vi "UHR-Fleezers Control (host) - 12.5.vi"() -> ()   [LabVIEW 2012] (continued)
            n2305 = Bundle("T1 Y", "T1 X", "T1 Sum", "T2 Y", "T2 X", "T2 Sum", "T1 FB X", "T1 FB Sum", "T2 FB X", "T2 FB Sum", "PSD Y", "PSD X", "PSD Y Sum") -> (w4151:T42)  [unwired: 1 out]
            n2306 = Cluster To Array(cluster=w4151) -> (array=w4160:string[])
          }
          frame "IR-QPD + PSD + FB-QPD XY positions" {
            w4225 = 4  # Channel pattern
            # "time average x2 the 3 psd signals (detection laser)"
            # "deinterlace 3 signals from qpds"
            n2307 = Decimate 1D Array(w4249) -> (w4248:i16[], w4247:i16[], w4226:i16[], w4246:i16[], w4192:i16[], w4238:i16[], w4237:i16[], w4214:i16[])
            n2308 = Decimate 1D Array "Feedback Sum"(w4226) -> (w4210:i16[], w4208:i16[])
            n2309 = Decimate 1D Array "QPD Y"(w4248) -> (w4245:i16[], w4228:i16[])
            n2310 = Decimate 1D Array "QPD X"(w4247) -> (w4244:i16[], w4242:i16[])
            n2311 = Decimate 1D Array "Feedback Y"(w4192) -> (w4191:i16[], w4190:i16[])
            n2312 = Decimate 1D Array "QPD Sum"(w4246) -> (w4243:i16[], w4241:i16[])
            n2313 = Decimate 1D Array "Feedback X"(w4214) -> (w4211:i16[], w4209:i16[])
            n2314 = call "downsample 1D array - double.vi"("Ave N"=2.0, "Array In"=w4238) -> ("Array Out"=w4213:dbl[])  [unwired: 1 out]
            n2315 = call "downsample 1D array - double.vi"("Ave N"=2.0, "Array In"=w4237) -> ("Array Out"=w4212:dbl[])  [unwired: 1 out]
            n2316 = Interleave 1D Arrays(w4245, w4244, w4243, w4228, w4242, w4241, w4191, w4211, w4210, w4190, w4209, w4208, w4213, w4212) -> (w4236:dbl[])
            n2317 = Divide(x=w4236, y=3276.7) -> (x/y=w4235:dbl[])
            n2318 = Decimate 1D Array(w4235) -> (w4234:dbl[], w4233:dbl[], w4232:dbl[], w4231:dbl[], w4230:dbl[], w4229:dbl[], w4187:dbl[], w4201:dbl[], w4185:dbl[], w4186:dbl[], w4199:dbl[], w4183:dbl[], w4197:dbl[], w4195:dbl[])
            n2319 = Negate(x=w4195) -> (-x=w4193:dbl[])
            n2320 = Divide(x=w4197, y=w4193) -> (x/y=w4196:dbl[])
            n2321 = Divide(x=w4186, y=w4183) -> (x/y=w4182:dbl[])
            n2322 = Divide(x=w4187, y=w4185) -> (x/y=w4184:dbl[])
            n2323 = Divide(x=w4234, y=w4232) -> (x/y=w4218:dbl[])
            n2324 = Divide(x=w4233, y=w4232) -> (x/y=w4217:dbl[])
            n2325 = Divide(x=w4231, y=w4229) -> (x/y=w4216:dbl[])
            n2326 = Divide(x=w4230, y=w4229) -> (x/y=w4215:dbl[])
            n2327 = Divide(x=w4201, y=w4185) -> (x/y=w4200:dbl[])
            n2328 = Divide(x=w4199, y=w4183) -> (x/y=w4198:dbl[])
            n2329 = Build Array(w4218, w4217, w4232, w4216, w4215, w4229, w4184, w4200, w4185, w4182, w4198, w4183, w4196, w4195) -> (w4194:dbl[][])
            n2330 = Bundle("T1 Y", "T1 X", "T1 Sum", "T2 Y", "T2 X", "T2 Sum", "T1 FB Y", "T1 FB X", "T1 FB Sum", "T2 FB Y", "T2 FB X", "T2 FB Sum", "PSD X", "PSD Y Sum") -> (w4181:T43)  [unwired: 1 out]
            n2331 = To Word Integer(number=w4236) -> (16bit integer=w4180:i16[])
            n2332 = Cluster To Array(cluster=w4181) -> (array=w4227:string[])
          }
        }
      }
    }
    "AI labels" <- w3250
    n2333 = local read "APD Integration Time (s)"() -> (w3223:dbl)
    n2334 = Array Size(array=w3265) -> (size(s)=w3310:i32)
    n2335 = call <vilib>:"Std Deviation and Variance.vi"("X"=w3212) -> ("standard deviation"=w3211:dbl)  [unwired: 1 in, 2 out]
    n2336 = Add Array Elements(numeric array=w3212) -> (sum=w3213:u32)
    n2337 = Add Array Elements(numeric array=w3265) -> (sum=w3320:u32)
    n2338 = call <vilib>:"Std Deviation and Variance.vi"("X"=w3265) -> ("standard deviation"=w3264:dbl)  [unwired: 1 in, 2 out]
    n2339 = Divide(x=w3211, y=w3053) -> (x/y=w3208:dbl)
    "Rate sigma (Hz) 2" <- w3208
    n2340 = Multiply(x=w3053, y=w3310) -> (x*y=w3055:dbl)
    "Int. Time (s)" <- w3055
    n2341 = Divide(x=w3213, y=w3055) -> (x/y=w3209:dbl)
    "APD 2 Rate (Hz)" <- w3209
    n2342 = Multiply(x="APD Disp. Scale", y=w3216) -> (x*y=w3225:waveform(dbl)[])
    n2343 = Divide(x=w3320, y=w3055) -> (x/y=w3262:dbl)
    "APD 1 Rate (Hz)" <- w3262
    n2344 = Divide(x=w3264, y=w3053) -> (x/y=w3263:dbl)
    "Rate sigma (Hz)" <- w3263
    n2345 = Divide(x=w3208, y=w3209) -> (x/y=→"Sigma/Mean 2":dbl)
    n2346 = Multiply(x="APD Disp. Downsample", y=w3223) -> (x*y=w3221:dbl)
    n2347 = Divide(x=w3263, y=w3262) -> (x/y=→"Sigma/Mean":dbl)
    n2348 = Divide(x=w3225, y=w3221) -> (x/y=w3045:waveform(dbl)[])
    n2349 = Index Array(array=w3045, index=0) -> (element=w3205:waveform(dbl))
    n2350 = Index Array(array=w3045, index=1) -> (element=w3203:waveform(dbl))
    n2351 = Index Array(array=w3045, index=2) -> (element=w3047:waveform(dbl))
    n2352 = Subtract(x=w3205, y="APD 1 Offset") -> (x-y=w3201:waveform(dbl))
    n2353 = Subtract(x=w3203, y="APD 2 Offset") -> (x-y=w3200:waveform(dbl))
    n2354 = Subtract(x=w3047, y="APD 3 Offset") -> (x-y=w3044:waveform(dbl))
    n2355 = Add Array Elements(numeric array=w3054) -> (sum=w3057:u32)
    n2356 = call <vilib>:"Std Deviation and Variance.vi"("X"=w3054) -> ("standard deviation"=w3056:dbl)  [unwired: 1 in, 2 out]
    n2357 = Build Array(w3201, w3200, w3044) -> (→"APD Chart":waveform(dbl)[])
    n2358 = Divide(x=w3057, y=w3055) -> (x/y=w3051:dbl)
    "APD 3 Rate (Hz)" <- w3051
    n2359 = Divide(x=w3056, y=w3053) -> (x/y=w3052:dbl)
    "Rate sigma (Hz) 3" <- w3052
    n2360 = Divide(x=w3052, y=w3051) -> (x/y=→"Sigma/Mean 3":dbl)
    n2361 = local read "Data Period (s)"() -> (w3108:dbl)
    n2362 = local read "BD 1 Frequency 2 (MHz)"() -> (w3141:dbl)
    n2363 = local read "BD 1 Frequency 1 (MHz)"() -> (w3142:dbl)
    n2364 = Decimate 1D Array(w3149) -> (w3173:i16[], w3172:i16[], w3170:i16[], w3169:i16[])  [unwired: 9 out]
    n2365 = Multiply(x=w3108, y="Trap Pos. Disp. Downsample") -> (x*y=w3106:dbl)
    n2366 = Divide(x=w3173, y=w3172) -> (x/y=w3174:dbl[])
    n2367 = Divide(x=w3170, y=w3169) -> (x/y=w3171:dbl[])
    n2368 = local read "AOM X Cal (nm/MHz)"() -> (w3139:dbl)
    n2369 = Split 1D Array(array=w3174, index="N El. to Ave.") -> (second subarray=w3177:dbl[])  [unwired: 1 out]
    n2370 = Split 1D Array(array=w3171, index="N El. to Ave.") -> (second subarray=w3176:dbl[])  [unwired: 1 out]
    n2371 = Multiply(x=w3108, y="Trap Disp. Downsample") -> (x*y=w3187:dbl)
    "Display Period (s)" <- w3187
    n2372 = for "Trap AI" {
      tunnel: [w3974] -> w3352 mode=indexing
      tunnel: w3185 -> [w3965]
      tunnel: "Trap Disp. Downsample" -> [w3972]
      tunnel: w3251 -> [w3970] mode=indexing
      tunnel: w3108 -> [w3969]
      tunnel: w3250 -> [w3968] mode=indexing
      tunnel: [w3967] -> w3220 mode=indexing
      tunnel: w3187 -> [w3966]
      workers-P: _ -> [_]
      n2373 = Bundle By Name("Y"=w3970, "dt"=w3969) -> (w3971:waveform(dbl))  [unwired: 1 out]
      n2374 = Set Waveform Attribute(5:w3968, 6:"NI_ChannelName" ("name"), 7:w3971) -> (3:w3967:waveform(dbl))  [unwired: 1 in, 2 out]
      n2375 = call "downsample 1D array - double.vi"("Ave N"=w3972, "Array In"=w3970) -> ("Array Out"=w3973:dbl[])  [unwired: 1 out]
      n2376 = Bundle By Name(cluster=w3967, "t0"=w3965, "Y"=w3973, "dt"=w3966) -> (w3974:waveform(dbl))
    }
    n2377 = Bundle("BD 1 Frequency 1 (MHz)"=w3142, "BD 1 Frequency 2 (MHz)"=w3141) -> (w3143:T44)  [unwired: 1 out]
    n2378 = call-poly <vilib>:"Mean.vi"("X"=w3176) -> ("mean"=w3164:dbl)  [unwired: 1 out]
    n2379 = call-poly <vilib>:"Mean.vi"("X"=w3177) -> ("mean"=w3165:dbl)  [unwired: 1 out]
    n2380 = Reciprocal(x=w3187) -> (1/x=→"Trap Disp. Freq. (Hz)":dbl)
    n2381 = Cluster To Array(cluster=w3143) -> (array=w3140:dbl[])
    n2382 = local read "Trap X AI1 (DMA)"() -> (w3175:T13)
    n2383 = local read "Data points/scans (MCL)"() -> (w3330:dbl)
    n2384 = To Fixed-Point(number=w3164) -> (fixed-point=w3162:fxp<+/-,16,1>)  [unwired: 1 in]
    n2385 = To Fixed-Point(number=w3165) -> (fixed-point=w3163:fxp<+/-,16,1>)  [unwired: 1 in]
    n2386 = Bundle("Trap 1 Pos.", "Trap 2 Pos.") -> (w3184:cluster{string, string})  [unwired: 1 out]
    n2387 = Bundle By Name(cluster=w3175, "Set 1"=w3163, "Set 2"=w3162) -> (→"Trap X AI1 (DMA)":T13)
    n2388 = Cluster To Array(cluster=w3184) -> (array=w3181:string[])
    n2389 = Unbundle(w3041) -> (w3042:u32[])  [unwired: 2 out]
    n2390 = Select(t=-1.0, s="Negate Y Axis", f=1.0) -> (s? t:f=w3125:dbl)
    n2391 = for "Trap Position" {
      tunnel: w3189 -> [w3560] mode=indexing
      tunnel: "Trap Pos. Disp. Downsample" -> [w3559]
      tunnel: w3106 -> [w3557]
      tunnel: w3185 -> [w3556]
      tunnel: w3181 -> [w3554] mode=indexing
      tunnel: [w3553] -> w3095 mode=indexing
      tunnel: w3140 -> [w3551] mode=indexing
      tunnel: w3139 -> [w3549]
      tunnel: w3125 -> [w3548]
      n2392 = call "downsample 1D array - double.vi"("Ave N"=w3559, "Array In"=w3560) -> ("Array Out"=w3558:dbl[])  [unwired: 1 out]
      n2393 = Subtract(x=w3558, y=w3551) -> (x-y=w3552:dbl[])
      n2394 = Multiply(x=w3549, y=w3552) -> (x*y=w3550:dbl[])
      n2395 = Multiply(x=w3548, y=w3550) -> (x*y=w3547:dbl[])
      n2396 = Bundle By Name("Y"=w3547, "dt"=w3557, "t0"=w3556) -> (w3555:waveform(dbl))  [unwired: 1 out]
      n2397 = Set Waveform Attribute(5:w3554, 6:"NI_ChannelName" ("name"), 7:w3555) -> (3:w3553:waveform(dbl))  [unwired: 1 in, 2 out]
    }
    n2398 = To Double Precision Float(number=w3042) -> (double precision float=w3248:dbl[])
    n2399 = local read "Display Period (s)"() -> (w3237:dbl)
    n2400 = Increment(x=w3330) -> (x+1=w3331:dbl)
    n2401 = Index Array(array=w3095, index=0) -> (element=w3099:waveform(dbl))
    n2402 = Index Array(array=w3095, index=1) -> (element=w3094:waveform(dbl))
    n2403 = feedback #7(w3331) -> (w3334:dbl)
    n2404 = Select(t=0, s=w3321, f=w3334) -> (s? t:f=w3327:dbl)
    n2405 = Array Size(array=w3248) -> (size(s)=w3333:i32)
    n2406 = Build Array (concatenate)(w3216, w3352) -> (w3218:waveform(dbl)[])
    "All Signals" <- w3218
    n2407 = Add(x=w3333, y=w3327) -> (x+y=w3328:dbl)
    n2408 = Unbundle By Name(w3099) -> ("Y"=w3100:dbl[])
    n2409 = Divide(x="Bead Sep. Int. Time (s)", y=w3237) -> (x/y=w3135:dbl)
    n2410 = Add(x=w3100, y="FB Trap Pos Offset") -> (x+y=w3098:dbl[])
    "T1 x pos data" <- w3098
    n2411 = Greater?(x=w3328, y=w3330) -> (0:w3329:bool)
    n2412 = feedback #8(w3098) -> (w3137:dbl[])
    n2413 = Build Array (concatenate)(w3098, w3137) -> (w3136:dbl[])
    n2414 = Bundle By Name(cluster=w3099, "Y"=w3098) -> (w3097:waveform(dbl))
    n2415 = Select(t=w3327, s=w3329, f=w3328) -> (s? t:f=w3326:dbl)
    n2416 = feedback-in #7(w3326) -> ()
    n2417 = local read "MCL Scanning"() -> (w3324:bool)
    n2418 = Bundle(w3097, w3094) -> (w3093:cluster{waveform(dbl), waveform(dbl)})  [unwired: 1 out]
    n2419 = Split 1D Array(array=w3136, index=w3135) -> (first subarray=w3129:dbl[])  [unwired: 1 out]
    n2420 = feedback-in #8(w3129) -> ()
    n2421 = Not(x=w3329) -> (.not. x?=w3323:bool)
    n2422 = Cluster To Array(cluster=w3093) -> (array=w3069:waveform(dbl)[])
    "Trap Positions" <- w3069
    n2423 = call-poly <vilib>:"Mean.vi"("X"=w3129) -> ("mean"=w3128:dbl)  [unwired: 1 out]
    "Mean T1 Position (nm)" <- w3128
    n2424 = Subtract(x=w3129, y=w3128) -> (x-y=w3134:dbl[])
    n2425 = Square(x=w3134) -> (x^2=w3133:dbl[])
    n2426 = And(x=w3323, y=w3324) -> (x .and. y?=w3325:bool)
    n2427 = call-poly <vilib>:"Mean.vi"("X"=w3133) -> ("mean"=w3132:dbl)  [unwired: 1 out]
    n2428 = Square Root(x=w3132) -> (sqrt(x)=w3131:dbl)
    n2429 = Or(x=w3325, y=w3321) -> (x .or. y?=w3322:bool)
    n2430 = Equal?(x="Tab Control 6", y=T34."High Res Display") -> (x = y?=w3254:bool)
    n2431 = Multiply(x=10.0, y=w3131) -> (x*y=→"Trap 1 Position RMS (A)":dbl)
    n2432 = case "For displaying the high resolution display (no downsampling)" shown="True" w3254 {
      tunnel: w3220 -> [_ w3580]
      frame False {
      }
      frame True {
        n2433 = Index Array(array=w3580, index="High Res. Display") -> (element=w3581:waveform(dbl))
        n2434 = call <vilib>:"Std Deviation and Variance.vi"("X"=w3581) -> ("mean"=w3588:dbl, "standard deviation"=w3593:dbl)  [unwired: 1 in, 1 out]
        "Mean Intensity" <- w3588
        "Sigma" <- w3593
        n2435 = Subtract(x=w3581, y=w3588) -> (x-y=w3587:waveform(dbl))
        n2436 = Select(t=w3587, s="Subtract mean", f=w3581) -> (s? t:f=→"1 Channel":waveform(dbl))
        n2437 = Divide(x=w3593, y=w3588) -> (x/y=→"Sigma/Mean":dbl)
        n2438 = feedback #9(1) -> (w3582:i32)
        n2439 = Greater Or Equal?(x=w3582, y="Slow mean N ave.") -> (x >= y?=w3595:bool)
        n2440 = Increment(x=w3582) -> (x+1=w3597:i32)
        n2441 = Select(t=1, s=w3595, f=w3597) -> (s? t:f=w3584:i32)
        n2442 = feedback-in #9(w3584) -> ()
        n2443 = feedback #10() -> (w3585:waveform(dbl))  [unwired: 1 out]
        n2444 = case shown="Default" w3582 {
          tunnel: [w3600 w3603] -> w3586
          tunnel: w3585 -> [w3602 _]
          tunnel: w3581 -> [w3601 w3603]
          frame Default {
            n2445 = call-poly <vilib>:"Append Waveforms.vi"("waveform B"=w3601, "waveform A"=w3602) -> ("waveform out"=w3600:waveform(dbl))  [unwired: 1 in, 8 out]
          }
          frame 1 {
          }
        }
        n2446 = feedback-in #10(w3586) -> ()
        n2447 = case shown="True" w3595 {
          tunnel: w3586 -> [_ w3599]
          frame False {
          }
          frame True {
            n2448 = call-poly <vilib>:"Mean.vi"("X"=w3599) -> ("mean"=→"Slow mean":dbl)  [unwired: 1 out]
          }
        }
      }
    }
    n2449 = case "For plotting results of scanning MCL (fluorescence and detection laser images)" shown="True" w3322 {
      tunnel: w3321 -> [_ w3712]
      tunnel: w3330 -> [_ _]
      tunnel: w3220 -> [_ w3842]
      tunnel: w3198 -> [_ w3750]
      tunnel: w3041 -> [_ w3719]
      frame False {
      }
      frame True {
        w3729 = u32 0 items=["Horizontal", "Vertical", "Central", "1st Diagonal", "2nd Diagonal"] ("Type of Symmetry")
        w3757 = u32 0 items=["Horizontal", "Vertical", "Central", "1st Diagonal", "2nd Diagonal"] ("Type of Symmetry")
        w3781 = u32 0 items=["Horizontal", "Vertical", "Central", "1st Diagonal", "2nd Diagonal"] ("Type of Symmetry")
        w3784 = u32 0 items=["Horizontal", "Vertical", "Central", "1st Diagonal", "2nd Diagonal"] ("Type of Symmetry")
        w3813 = u32 0 items=["Horizontal", "Vertical", "Central", "1st Diagonal", "2nd Diagonal"] ("Type of Symmetry")
        n2450 = Unbundle(w3719) -> (w3718:u32[], w3716:u32[], w3714:u32[])
        n2451 = To Double Precision Float(number=w3718) -> (double precision float=w3717:dbl[])
        n2452 = To Double Precision Float(number=w3716) -> (double precision float=w3715:dbl[])
        n2453 = To Double Precision Float(number=w3714) -> (double precision float=w3713:dbl[])
        n2454 = Index Array(array=w3842, index=10) -> (element=w3848:waveform(dbl))
        n2455 = Index Array(array=w3842, index=11) -> (element=w3845:waveform(dbl))
        n2456 = local read "Cycles/step (MCL)"() -> (w3798:u64)
        n2457 = Index Array(array=w3842, index="Channel") -> (element=w3844:waveform(dbl))
        n2458 = Unbundle(w3750) -> ("New Image"=w3749:T2, "New Image"=w3748:T2, "New Image"=w3720:T2, "New Image"=w3721:T2, "New Image"=w3722:T2)
        n2459 = local read "Scan steps (MCL)"() -> (w3708:u64)
        n2460 = Unbundle By Name(w3848) -> ("Y"=w3800:dbl[])
        n2461 = Unbundle By Name(w3845) -> ("Y"=w3802:dbl[])
        n2462 = local read "Scan lines (y)"() -> (w3709:u64)
        n2463 = local read "N APD Samp/step"() -> (w3711:dbl)
        n2464 = Unbundle By Name(w3844) -> ("Y"=w3807:dbl[])
        n2465 = call "downsample 1D array - double.vi"("Ave N"=w3798, "Array In"=w3800) -> ("Array Out"=w3799:dbl[])  [unwired: 1 out]
        n2466 = call "downsample 1D array - double.vi"("Ave N"=w3798, "Array In"=w3802) -> ("Array Out"=w3801:dbl[])  [unwired: 1 out]
        n2467 = call "downsample 1D array - double.vi"("Ave N"=w3798, "Array In"=w3807) -> ("Array Out"=w3806:dbl[])  [unwired: 1 out]
        n2468 = Multiply(x=w3708, y=u64 2) -> (x*y=w3710:u64)
        n2469 = feedback #11(w3715) -> (w3775:dbl[])
        n2470 = Build Array (concatenate)(w3775, w3715) -> (w3774:dbl[])
        n2471 = feedback #12(w3713) -> (w3747:dbl[])
        n2472 = Build Array (concatenate)(w3747, w3713) -> (w3746:dbl[])
        n2473 = Select(t=w3715, s=w3712, f=w3774) -> (s? t:f=w3759:dbl[])
        n2474 = feedback-in #11(w3759) -> ()
        n2475 = Select(t=w3713, s=w3712, f=w3746) -> (s? t:f=w3731:dbl[])
        n2476 = feedback-in #12(w3731) -> ()
        n2477 = feedback #13(w3717) -> (w3868:dbl[])
        n2478 = Build Array (concatenate)(w3868, w3717) -> (w3850:dbl[])
        n2479 = Select(t=w3717, s=w3712, f=w3850) -> (s? t:f=w3854:dbl[])
        n2480 = feedback-in #13(w3854) -> ()
        n2481 = feedback #14(w3799) -> (w3856:dbl[])
        n2482 = Build Array (concatenate)(w3856, w3799) -> (w3847:dbl[])
        n2483 = feedback #15(w3806) -> (w3866:dbl[])
        n2484 = Build Array (concatenate)(w3866, w3806) -> (w3865:dbl[])
        n2485 = feedback #16(w3801) -> (w3858:dbl[])
        n2486 = Build Array (concatenate)(w3858, w3801) -> (w3859:dbl[])
        n2487 = Select(t=w3799, s=w3712, f=w3847) -> (s? t:f=w3803:dbl[])
        n2488 = feedback-in #14(w3803) -> ()
        n2489 = Select(t=w3806, s=w3712, f=w3865) -> (s? t:f=w3805:dbl[])
        n2490 = feedback-in #15(w3805) -> ()
        n2491 = Select(t=w3801, s=w3712, f=w3859) -> (s? t:f=w3804:dbl[])
        n2492 = feedback-in #16(w3804) -> ()
        n2493 = call "integrate 1D array interval - double.vi"("Ave N"=w3711, "Array In"=w3759) -> ("Array Out"=w3770:dbl[])  [unwired: 1 out]
        n2494 = call "integrate 1D array interval - double.vi"("Ave N"=w3711, "Array In"=w3731) -> ("Array Out"=w3742:dbl[])  [unwired: 1 out]
        n2495 = call "integrate 1D array interval - double.vi"("Ave N"=w3711, "Array In"=w3854) -> ("Array Out"=w3853:dbl[])  [unwired: 1 out]
        n2496 = Array Size(array=w3770) -> (size(s)=w3771:i32)
        n2497 = Array Size(array=w3742) -> (size(s)=w3743:i32)
        n2498 = Array Size(array=w3853) -> (size(s)=w3855:i32)
        n2499 = Multiply(x=w3709, y=w3710) -> (x*y=w3773:u64)
        n2500 = Multiply(x=w3709, y=w3710) -> (x*y=w3745:u64)
        n2501 = Multiply(x=w3709, y=w3710) -> (x*y=w3863:u64)
        n2502 = Subtract(x=w3773, y=w3771) -> (x-y=w3764:u64)
        n2503 = call-poly <vilib>:"Mean.vi"("X"=w3770) -> ("mean"=w3761:dbl)  [unwired: 1 out]
        n2504 = Subtract(x=w3745, y=w3743) -> (x-y=w3736:u64)
        n2505 = call-poly <vilib>:"Mean.vi"("X"=w3742) -> ("mean"=w3733:dbl)  [unwired: 1 out]
        n2506 = Subtract(x=w3863, y=w3855) -> (x-y=w3797:u64)
        n2507 = call-poly <vilib>:"Mean.vi"("X"=w3853) -> ("mean"=w3794:dbl)  [unwired: 1 out]
        n2508 = call-poly <vilib>:"Mean.vi"("X"=w3803) -> ("mean"=w3787:dbl)  [unwired: 1 out]
        n2509 = call-poly <vilib>:"Mean.vi"("X"=w3805) -> ("mean"=w3792:dbl)  [unwired: 1 out]
        n2510 = call-poly <vilib>:"Mean.vi"("X"=w3804) -> ("mean"=w3790:dbl)  [unwired: 1 out]
        n2511 = Initialize Array(1.0 ("element"), w3764) -> (w3760:dbl[])
        n2512 = Initialize Array(1.0 ("element"), w3736) -> (w3732:dbl[])
        n2513 = Initialize Array(1.0 ("element"), w3797) -> (w3788:dbl[])
        n2514 = Multiply(x=w3760, y=w3761) -> (x*y=w3762:dbl[])
        n2515 = Multiply(x=w3732, y=w3733) -> (x*y=w3734:dbl[])
        n2516 = Multiply(x=w3788, y=w3794) -> (x*y=w3795:dbl[])
        n2517 = Multiply(x=w3788, y=w3790) -> (x*y=w3791:dbl[])
        n2518 = Multiply(x=w3788, y=w3792) -> (x*y=w3793:dbl[])
        n2519 = Multiply(x=w3788, y=w3787) -> (x*y=w3789:dbl[])
        n2520 = Build Array (concatenate)(w3770, w3762) -> (w3772:dbl[])
        n2521 = Build Array (concatenate)(w3742, w3734) -> (w3744:dbl[])
        n2522 = Build Array (concatenate)(w3853, w3795) -> (w3862:dbl[])
        n2523 = Build Array (concatenate)(w3803, w3789) -> (w3857:dbl[])
        n2524 = Build Array (concatenate)(w3805, w3793) -> (w3861:dbl[])
        n2525 = Build Array (concatenate)(w3804, w3791) -> (w3860:dbl[])
        n2526 = Reshape Array(w3772, w3709, w3710) -> (w3768:dbl[][])
        n2527 = Reshape Array(w3744, w3709, w3710) -> (w3740:dbl[][])
        n2528 = Reshape Array(w3862, w3709, w3710) -> (w3840:dbl[][])
        n2529 = Reshape Array(w3857, w3709, w3710) -> (w3823:dbl[][])
        n2530 = Reshape Array(w3861, w3709, w3710) -> (w3815:dbl[][])
        n2531 = Reshape Array(w3860, w3709, w3710) -> (w3830:dbl[][])
        n2532 = Array Subset(array=w3768, index (col)=0 ("index"), length (col)=w3708) -> (w3767:dbl[][])  [unwired: 2 in]
        n2533 = Array Subset(array=w3768, index (col)=w3708) -> (w3765:dbl[][])  [unwired: 3 in]
        n2534 = Array Subset(array=w3740, index (col)=0 ("index"), length (col)=w3708) -> (w3739:dbl[][])  [unwired: 2 in]
        n2535 = Array Subset(array=w3740, index (col)=w3708) -> (w3737:dbl[][])  [unwired: 3 in]
        n2536 = Array Subset(array=w3830, index (col)=0 ("index"), length (col)=w3708) -> (w3835:dbl[][])  [unwired: 2 in]
        n2537 = Array Subset(array=w3830, index (col)=w3708) -> (w3833:dbl[][])  [unwired: 3 in]
        n2538 = Array Subset(array=w3840, index (col)=0 ("index"), length (col)=w3708) -> (w3839:dbl[][])  [unwired: 2 in]
        n2539 = Array Subset(array=w3840, index (col)=w3708) -> (w3837:dbl[][])  [unwired: 3 in]
        n2540 = Array Subset(array=w3815, index (col)=0 ("index"), length (col)=w3708) -> (w3821:dbl[][])  [unwired: 2 in]
        n2541 = Array Subset(array=w3815, index (col)=w3708) -> (w3819:dbl[][])  [unwired: 3 in]
        n2542 = Array Subset(array=w3823, index (col)=0 ("index"), length (col)=w3708) -> (w3828:dbl[][])  [unwired: 2 in]
        n2543 = Array Subset(array=w3823, index (col)=w3708) -> (w3826:dbl[][])  [unwired: 3 in]
        n2544 = for {
          tunnel: w3767 -> [w3872] mode=indexing
          tunnel: [w3871] -> w3766 mode=indexing
          workers-P: _ -> [_]
          n2545 = Reverse 1D Array(array=w3872) -> (reversed array=w3871:dbl[])
        }
        n2546 = for {
          tunnel: w3739 -> [w3870] mode=indexing
          tunnel: [w3869] -> w3738 mode=indexing
          workers-P: _ -> [_]
          n2547 = Reverse 1D Array(array=w3870) -> (reversed array=w3869:dbl[])
        }
        n2548 = for {
          tunnel: w3835 -> [w3878] mode=indexing
          tunnel: [w3877] -> w3834 mode=indexing
          workers-P: _ -> [_]
          n2549 = Reverse 1D Array(array=w3878) -> (reversed array=w3877:dbl[])
        }
        n2550 = for {
          tunnel: w3839 -> [w3880] mode=indexing
          tunnel: [w3879] -> w3838 mode=indexing
          workers-P: _ -> [_]
          n2551 = Reverse 1D Array(array=w3880) -> (reversed array=w3879:dbl[])
        }
        n2552 = for {
          tunnel: w3821 -> [w3874] mode=indexing
          tunnel: [w3873] -> w3820 mode=indexing
          workers-P: _ -> [_]
          n2553 = Reverse 1D Array(array=w3874) -> (reversed array=w3873:dbl[])
        }
        n2554 = for {
          tunnel: w3828 -> [w3876] mode=indexing
          tunnel: [w3875] -> w3827 mode=indexing
          workers-P: _ -> [_]
          n2555 = Reverse 1D Array(array=w3876) -> (reversed array=w3875:dbl[])
        }
        n2556 = Index Array(array=w3840, index (row)=0) -> (element=→"Waveform Graph":dbl[])  [unwired: 1 in]
        n2557 = Add(x=w3766, y=w3765) -> (x+y=w3752:dbl[][])
        n2558 = Add(x=w3738, y=w3737) -> (x+y=w3724:dbl[][])
        n2559 = Add(x=w3834, y=w3833) -> (x+y=w3832:dbl[][])
        n2560 = Add(x=w3838, y=w3837) -> (x+y=w3812:dbl[][])
        n2561 = Add(x=w3820, y=w3819) -> (x+y=w3818:dbl[][])
        n2562 = Add(x=w3827, y=w3826) -> (x+y=w3825:dbl[][])
        n2563 = Divide(x=w3818, y=2) -> (x/y=w3816:dbl[][])
        n2564 = Divide(x=w3832, y=2) -> (x/y=w3777:dbl[][])
        n2565 = To Single Precision Float(number=w3812) -> (single precision float=w3811:sgl[][])
        n2566 = To Single Precision Float(number=w3752) -> (single precision float=w3756:sgl[][])
        n2567 = To Single Precision Float(number=w3724) -> (single precision float=w3728:sgl[][])
        n2568 = Divide(x=w3825, y=2) -> (x/y=w3779:dbl[][])
        n2569 = Transpose 2D Array(2D array=w3816) -> (transposed array=→"Data map":dbl[][])
        n2570 = To Single Precision Float(number=w3777) -> (single precision float=w3783:sgl[][])
        n2571 = To Single Precision Float(number=w3779) -> (single precision float=w3780:sgl[][])
        n2572 = call "IMAQ ArrayToImage"("Image Pixels (Float)"=w3811, "Image"=w3749) -> ("Image Out"=w3814:T2)  [unwired: 8 in, 1 out]
        n2573 = call "IMAQ ArrayToImage"("Image Pixels (Float)"=w3756, "Image"=w3748) -> ("Image Out"=w3758:T2)  [unwired: 8 in, 1 out]
        n2574 = call "IMAQ ArrayToImage"("Image Pixels (Float)"=w3728, "Image"=w3720) -> ("Image Out"=w3730:T2)  [unwired: 8 in, 1 out]
        n2575 = call "IMAQ ArrayToImage"("Image Pixels (Float)"=w3783, "Image"=w3721) -> ("Image Out"=w3785:T2)  [unwired: 8 in, 1 out]
        n2576 = call "IMAQ Symmetry"("Type of Symmetry"=w3813, "Image Src"=w3814) -> ("Image Dst Out"=w3809:T2)  [unwired: 3 in, 1 out]
        n2577 = call "IMAQ ArrayToImage"("Image Pixels (Float)"=w3780, "Image"=w3722) -> ("Image Out"=w3782:T2)  [unwired: 8 in, 1 out]
        n2578 = call "IMAQ Symmetry"("Type of Symmetry"=w3757, "Image Src"=w3758) -> ("Image Dst Out"=w3754:T2)  [unwired: 3 in, 1 out]
        n2579 = call "IMAQ Symmetry"("Type of Symmetry"=w3729, "Image Src"=w3730) -> ("Image Dst Out"=w3726:T2)  [unwired: 3 in, 1 out]
        n2580 = call "IMAQ Symmetry"("Type of Symmetry"=w3784, "Image Src"=w3785) -> ("Image Dst Out"=→"Detection Laser X":T2)  [unwired: 3 in, 1 out]
        n2581 = call "IMAQ Symmetry"("Type of Symmetry"=w3781, "Image Src"=w3782) -> ("Image Dst Out"=→"Detection Laser Y":T2)  [unwired: 3 in, 1 out]
        n2582 = call "IMAQ Set Simple Calibration"("Calibration Axis Info"=T35 {"Origin Pixel"={"X"=0.0, "Y"=0.0}, "Angle Relative to Horizontal (deg)"=0.0, "Axis Reference"=0}, "Grid Descriptor"=T36 {"X Step"=0.3, "Y Step"=0.3, "Unit"=enum."Undefined"}, "Image"=w3809) -> ("Calibrated Image"=→"APD 1":T2)  [unwired: 7 in, 1 out]
        n2583 = call "IMAQ Set Simple Calibration"("Calibration Axis Info"=T35 {"Origin Pixel"={"X"=0.0, "Y"=0.0}, "Angle Relative to Horizontal (deg)"=0.0, "Axis Reference"=0}, "Grid Descriptor"=T36 {"X Step"=0.3, "Y Step"=0.3, "Unit"=enum."Undefined"}, "Image"=w3754) -> ("Calibrated Image"=→"APD 2":T2)  [unwired: 7 in, 1 out]
        n2584 = call "IMAQ Set Simple Calibration"("Calibration Axis Info"=T35 {"Origin Pixel"={"X"=0.0, "Y"=0.0}, "Angle Relative to Horizontal (deg)"=0.0, "Axis Reference"=0}, "Grid Descriptor"=T36 {"X Step"=0.3, "Y Step"=0.3, "Unit"=enum."Undefined"}, "Image"=w3726) -> ("Calibrated Image"=→"APD 3":T2)  [unwired: 7 in, 1 out]
      }
    }
    n2585 = case "For computing FFTs for display" shown="True" "Compute FFT" {
      tunnel: w3220 -> [_ w4352]
      frame False {
      }
      frame True {
        n2586 = Build Array("FFT 1 Choice 1", "FFT 1 Choice 2", "FFT 2 Choice 1", "FFT 2 Choice 2") -> (w4345:u16[])
        n2587 = Array Size(array=w4352) -> (size(s)=w4351:i32)
        n2588 = feedback-in #17(w4345) -> ()
        n2589 = feedback #17(u16[] [100, 100, 100, 100]) -> (w4346:u16[])
        n2590 = feedback-in #18("# Spectra to Ave.") -> ()
        n2591 = feedback #18("# Spectra to Ave.") -> (w4343:dbl)
        n2592 = Not Equal?(x="# Spectra to Ave.", y=w4343) -> (x != y?=w4342:bool)
        n2593 = Not Equal?(x=w4345, y=w4346) -> (x != y?=w4344:bool)
        n2594 = feedback #19(1.0) -> (w4329:dbl)
        n2595 = Compound Arithmetic op=OR("Reset FFT", w4344, w4342) -> (w4327:bool)
        n2596 = Select(t=1.0, s=w4327, f=w4329) -> (s? t:f=w4331:dbl)
        n2597 = Greater?(x=w4331, y="# Spectra to Ave.") -> (0:w4350:bool)
        n2598 = Increment(x=w4331) -> (x+1=w4330:dbl)
        n2599 = feedback-in #19(w4330) -> ()
        n2600 = local read "DMA Update Period (s)"() -> (w4325:dbl)
        n2601 = Multiply(x="# Spectra to Ave.", y=w4325) -> (x*y=→"Ave. Time (s)":dbl)
        n2602 = Build Array(cluster{"f0":dbl, "df":dbl, "magnitude":dbl[]} {"f0"=0.0, "df"=0.0, "magnitude"=[]} ("PSD")) -> (w4334:cluster{"f0":dbl, "df":dbl, "magnitude":dbl[]}[])
        n2603 = Build Array(w4334, w4334, w4334, w4334) -> (w4336:T45)
        n2604 = feedback #20(w4336) -> (w4341:T45)
        n2605 = for {
          N: 4 -> [_]
          tunnel: w4345 -> [w4374] mode=indexing
          tunnel: w4352 -> [w4375]
          tunnel: w4351 -> [w4377]
          tunnel: w4327 -> [w4370]
          tunnel: w4350 -> [w4369]
          tunnel: "# Spectra to Ave." -> [w4368]
          tunnel: [w4367] -> w4340 mode=indexing
          tunnel: w4341 -> [w4372] mode=indexing
          tunnel: [w4371] -> w4328 mode=indexing
          tunnel: w4331 -> [w4366]
          n2606 = Less?(x=w4374, y=w4377) -> (x < y?=w4376:bool)
          n2607 = Index Array(array=w4375, index=w4374) -> (element=w4373:waveform(dbl))
          n2608 = case shown="True" w4376 {
            tunnel: w4373 -> [_ w4394]
            tunnel: w4372 -> [w4379 w4392]
            tunnel: [w4379 w4380] -> w4371
            tunnel: w4370 -> [_ w4391]
            tunnel: w4369 -> [_ w4384]
            tunnel: w4368 -> [_ w4383]
            tunnel: [cluster{"f0":dbl, "df":dbl, "magnitude":dbl[]} {"f0"=0.0, "df"=0.0, "magnitude"=[]} ("PSD") w4385] -> w4367
            tunnel: w4366 -> [_ w4382]
            frame False {
            }
            frame True {
              n2609 = call <vilib>:"Std Deviation and Variance.vi"("X"=w4394) -> ("mean"=w4395:dbl)  [unwired: 1 in, 2 out]
              n2610 = Subtract(x=w4394, y=w4395) -> (x-y=w4393:waveform(dbl))
              n2611 = xnode "Spectral Measurements"("Signals"=w4393) -> ("PSD"=w4387:cluster{"f0":dbl, "df":dbl, "magnitude":dbl[]})  [unwired: 1 in, 1 out]
              n2612 = case shown="False" w4391 {
                tunnel: w4392 -> [w4404 _]
                tunnel: [w4400 w4409] -> w4380
                tunnel: w4387 -> [w4403 w4410]
                tunnel: w4384 -> [w4402 _]
                frame False {
                  n2613 = Build Array (concatenate)(w4404, w4403) -> (w4401:cluster{"f0":dbl, "df":dbl, "magnitude":dbl[]}[])
                  n2614 = case shown="True" w4402 {
                    tunnel: w4401 -> [w4405 w4408]
                    tunnel: [w4405 w4406] -> w4400
                    frame False {
                    }
                    frame True {
                      n2615 = Delete From Array(array=w4408, index=0) -> (array with subset deleted=w4406:cluster{"f0":dbl, "df":dbl, "magnitude":dbl[]}[])  [unwired: 1 in, 1 out]
                    }
                  }
                }
                frame True {
                  n2616 = Build Array(w4410) -> (w4409:cluster{"f0":dbl, "df":dbl, "magnitude":dbl[]}[])
                }
              }
              n2617 = for {
                tunnel: w4380 -> [w4399] mode=indexing
                tunnel: [w4398] -> w4390 mode=indexing
                workers-P: _ -> [_]
                n2618 = Unbundle By Name(w4399) -> ("magnitude"=w4398:dbl[])
              }
              n2619 = Transpose 2D Array(2D array=w4390) -> (transposed array=w4389:dbl[][])
              n2620 = for {
                tunnel: w4389 -> [w4397] mode=indexing
                tunnel: [w4396] -> w4388 mode=indexing
                workers-P: _ -> [_]
                n2621 = Add Array Elements(numeric array=w4397) -> (sum=w4396:dbl)
              }
              n2622 = Select(t=w4383, s=w4384, f=w4382) -> (s? t:f=w4381:dbl)
              n2623 = Divide(x=w4388, y=w4381) -> (x/y=w4386:dbl[])
              n2624 = Bundle By Name(cluster=w4387, "magnitude"=w4386) -> (w4385:cluster{"f0":dbl, "df":dbl, "magnitude":dbl[]})
            }
          }
        }
        n2625 = case shown="True" w4327 {
          tunnel: w4328 -> [w4359 w4365]
          tunnel: [w4359 w4360] -> w4326
          frame False {
          }
          frame True {
            n2626 = Array Subset(array=w4365, index (row)=0 ("index"), length (row)=4 ("length"), index (col)=0 ("index"), length (col)=1 ("length")) -> (w4360:T45)
          }
        }
        n2627 = feedback-in #20(w4326) -> ()
        n2628 = Split 1D Array(array=w4340, index=2) -> (first subarray=→"FFT 1":cluster{"f0":dbl, "df":dbl, "magnitude":dbl[]}[], second subarray=→"FFT 2":cluster{"f0":dbl, "df":dbl, "magnitude":dbl[]}[])
      }
    }
    n2629 = Index Array(array=w3218, index=4) -> (element=w3274:waveform(dbl))
    n2630 = Index Array(array=w3218, index=7) -> (element=w3271:waveform(dbl))
    n2631 = Divide(x="T1 offset_x (mV)", y=1000.0) -> (x/y=w3275:dbl)
    n2632 = feedback-in #21("Calibration") -> ()
    n2633 = feedback #21(u16 1 ("Calibration")) -> (w3293:u16)
    n2634 = Divide(x="T2 offset_x (mV)", y=1000.0) -> (x/y=w3273:dbl)
    n2635 = case shown="2" "Calibration" {
      tunnel: "T1 alpha_x (nm/V)" -> [_ w3673 w3694]
      tunnel: "T1 kappa_x (pN/nm)" -> [_ _ w3684]
      tunnel: "T2 alpha_x (nm/V)" -> [_ w3672 w3692]
      tunnel: "T2 kappa_x (pN/nm)" -> [_ _ w3685]
      tunnel: w3274 -> [w3655 w3670 w3690]
      tunnel: w3271 -> [w3654 w3668 w3688]
      tunnel: [w3655 w3667 w3687] -> w3302
      tunnel: [w3654 w3666 w3686] -> w3301
      tunnel: ["T1 X (V)" ("Label.Text") "T1 X (nm)" ("Label.Text") "T1 X (pN)" ("Label.Text")] -> w3290
      tunnel: ["T2 X (V)" ("Label.Text") "T2 X (nm)" ("Label.Text") "T2 X (pN)" ("Label.Text")] -> w3289
      tunnel: ["Position (V)" ("Label.Text") "Position (nm)" ("Label.Text") "Force (pN)" ("Label.Text")] -> w3291
      tunnel: w3273 -> [_ w3658 w3677]
      tunnel: w3275 -> [_ w3661 w3679]
      tunnel: ["Mean (V)" ("Label.Text") "Mean (nm)" ("Label.Text") "Mean (pN)" ("Label.Text")] -> w3286
      tunnel: ["Difference (V)" ("Label.Text") "Difference (nm)" ("Label.Text") "Difference (pN)" ("Label.Text")] -> w3226
      frame 0, Default {
      }
      frame 1 {
        n2636 = Unbundle By Name(w3670) -> ("Y"=w3674:dbl[])
        n2637 = Unbundle By Name(w3668) -> ("Y"=w3659:dbl[])
        n2638 = Subtract(x=w3674, y=w3661) -> (x-y=w3662:dbl[])
        n2639 = Subtract(x=w3659, y=w3658) -> (x-y=w3660:dbl[])
        n2640 = Multiply(x=w3660, y=w3672) -> (x*y=w3669:dbl[])
        n2641 = Multiply(x=w3673, y=w3662) -> (x*y=w3671:dbl[])
        n2642 = Bundle By Name(cluster=w3668, "Y"=w3669) -> (w3666:waveform(dbl))
        n2643 = Bundle By Name(cluster=w3670, "Y"=w3671) -> (w3667:waveform(dbl))
      }
      frame 2 {
        n2644 = Unbundle By Name(w3690) -> ("Y"=w3695:dbl[])
        n2645 = Unbundle By Name(w3688) -> ("Y"=w3693:dbl[])
        n2646 = Subtract(x=w3693, y=w3677) -> (x-y=w3678:dbl[])
        n2647 = Subtract(x=w3695, y=w3679) -> (x-y=w3680:dbl[])
        n2648 = Compound Arithmetic op=MULTIPLY(w3678, w3692, w3685) -> (w3689:dbl[])
        n2649 = Compound Arithmetic op=MULTIPLY(w3684, w3694, w3680) -> (w3691:dbl[])
        n2650 = Bundle By Name(cluster=w3688, "Y"=w3689) -> (w3686:waveform(dbl))
        n2651 = Bundle By Name(cluster=w3690, "Y"=w3691) -> (w3687:waveform(dbl))
      }
    }
    n2652 = case shown="True" "Read Lateness and Rel Phase" {
      tunnel: w3092 -> [w3604 w3643]
      tunnel: w3091 -> [w3605 w3642]
      tunnel: [w3604 w3609] -> w3268
      tunnel: [w3605 w3608] -> w3267
      frame False {
      }
      frame True {
        n2653 = xnode "Read/Write Control"("FPGA VI Reference In"=w3643, "error in"=w3642) -> ("FPGA VI Reference Out"=w3611:T20, "error out"=w3610:errorcluster, "GI Relative phase"=→"GI relative phase":i16, "Relative phase"=→"Relative phase (AI1)":i16, "AI Late Counter"=→"Late Counter (AI1)":u8, "GI Late Counter"=→"GI Late Counter":u8, "MCL Late Counter"=→"MCL Late Counter":u8, "MCL Relative Phase"=→"Relative Phase (MCL)":i16, "APD Acq Relative Phase"=→"APD Acq Relative Phase":i16, "APD 1 Gate Relative Phase"=→"APD 1 Gate Relative Phase":i16, "APD 2 Gate Relative Phase"=→"APD 2 Gate Relative Phase":i16, "APD Acq Late Counter"=→"APD Acq Late Counter":u8, "APD 1 Gate Late Counter"=→"APD 1 Gate Late Counter":u8, "APD 2 Gate Late Counter"=→"APD 2 Gate Late Counter":u8, "Green FB Relative Phase"=→"Relative phase (Green FB)":i16, "GI Relative phase 2"=→"GI relative phase 2":i16, "GI Late Counter 2"=→"GI Late Counter 2":u8, "Trap Pos FIFO Timeout"=→"Trap Pos FIFO Timeout":u16, "Trap AI FIFO Timeout"=→"Trap AI FIFO Timeout":u16, "RI Late Counter"=→"RI Late Counter":u8, "RI Late Counter 2"=→"RI Late Counter 2", "RI Relative phase"=→"RI relative phase":i16, "RI Relative phase 2"=→"RI relative phase 2", "Red FB Relative Phase"=→"Relative phase (RI FB)", "Red Late Counter"=→"Red AI Late Counter", "Green Late Counter"=→"Green AI Late Counter":u8, "BI Late Counter (AO)"=→"Late Counter (BI AO)":u8, "Blue Late Counter (D)"=→"Late Counter (BI DO)":u8, "Blue Int Late Counter"=→"Late Counter (BI AI)", "Blue Int Relative Phase"=→"Relative phase (BI AI)", "BI Relative phase (AO)"=→"Relative phase (BI AO)":i16, "BI Relative phase (D)"=→"Relative phase (BI DO)":i16)
        n2654 = xnode "Read/Write Control"("FPGA VI Reference In"=w3611, "error in"=w3610) -> ("FPGA VI Reference Out"=w3609:T20, "error out"=w3608:errorcluster, "APD 3 Gate Late Counter"=→"APD 3 Gate Late Counter":u8, "APD 3 Gate Relative Phase"=→"APD 3 Gate Relative Phase":i16)
      }
    }
    n2655 = Not Equal?(x=w3293, y="Calibration") -> (x != y?=w3252:bool)
    n2656 = case shown="True" w3252 {
      tunnel: w3291 -> [_ w3648]
      tunnel: w3290 -> [_ w3647]
      tunnel: w3289 -> [_ w3646]
      tunnel: w3286 -> [_ w3645]
      tunnel: w3226 -> [_ w3644]
      frame False {
      }
      frame True {
        n2657 = property on="Force" class="WFChart (strict)"("YScale.NameLbl.Text"=w3648) -> ()  [unwired: 2 in, 2 out]
        n2658 = property on="T2 X" class="DigNum (strict)"("Caption.Text"=w3646) -> ()  [unwired: 2 in, 2 out]
        n2659 = property on="T1 X" class="DigNum (strict)"("Caption.Text"=w3647) -> ()  [unwired: 2 in, 2 out]
        n2660 = property on="Mean" class="DigNum (strict)"("Caption.Text"=w3645) -> ()  [unwired: 2 in, 2 out]
        n2661 = property on="Difference" class="DigNum (strict)"("Caption.Text"=w3644) -> ()  [unwired: 2 in, 2 out]
      }
    }
    n2662 = Unbundle By Name(w3274) -> ("Y"=w3277:dbl[])
    n2663 = Unbundle By Name(w3271) -> ("Y"=w3280:dbl[])
    n2664 = Subtract(x=w3277, y=w3275) -> (x-y=w3278:dbl[])
    n2665 = Subtract(x=w3280, y=w3273) -> (x-y=w3279:dbl[])
    n2666 = Multiply(x=w3279, y="T2 alpha_x (nm/V)") -> (x*y=w3074:dbl[])
    n2667 = Multiply(x="T1 alpha_x (nm/V)", y=w3278) -> (x*y=w3075:dbl[])
    n2668 = Not(x="Trap Trig. Fl.") -> (.not. x?=w3111:bool)
    n2669 = Multiply(x=w3301, y=-1.0) -> (x*y=w3282:waveform(dbl))
    n2670 = Subtract(x=w3075, y=w3074) -> (x-y=w3270:dbl[])
    n2671 = Unbundle By Name(w3301) -> ("Y"=w3242:dbl[])
    n2672 = Unbundle By Name(w3302) -> ("Y"=w3076:dbl[])
    n2673 = Negate(x=w3270) -> (-x=w3072:dbl[])
    n2674 = Build Array(w3302, w3282) -> (→"Force":waveform(dbl)[])
    n2675 = Subtract(x=w3072, y="Offset (nm)") -> (x-y=w3240:dbl[])
    n2676 = call-poly <vilib>:"Mean.vi"("X"=w3242) -> ("mean"=w3078:dbl)  [unwired: 1 out]
    "T2 X" <- w3078
    n2677 = Negate(x=w3242) -> (-x=w3243:dbl[])
    n2678 = call-poly <vilib>:"Mean.vi"("X"=w3076) -> ("mean"=w3079:dbl)  [unwired: 1 out]
    "T1 X" <- w3079
    n2679 = Negate(x=w3078) -> (-x=w3077:dbl)
    n2680 = Bundle By Name(cluster=w3274, "Y"=w3240) -> (w3217:waveform(dbl))
    "Bead Separation" <- w3217
    n2681 = Add(x=w3076, y=w3243) -> (x+y=w3244:dbl[])
    n2682 = Add(x=w3079, y=w3077) -> (x+y=w3288:dbl)
    n2683 = Subtract(x=w3079, y=w3077) -> (x-y=→"Difference":dbl)
    n2684 = Divide(x=w3244, y=2.0) -> (x/y=→"Vec Mean of T1 T2":dbl[])
    n2685 = Divide(x=w3288, y=2.0) -> (x/y=w3246:dbl)
    "Mean" <- w3246
    n2686 = feedback-in #22("Trap Trig. Fl.") -> ()
    n2687 = feedback #22("Trap Trig. Fl.") -> (w3109:bool)
    n2688 = And(x=w3111, y=w3109) -> (x .and. y?=w3110:bool)
    n2689 = case "If have just turned off triggering" shown="True" w3110 {
      tunnel: w3092 -> [_ w3439]
      tunnel: w3091 -> [_ w3438]
      frame False {
      }
      frame True {
        w3437 = FALSE ("FPGA Trap Trig")
        n2690 = xnode "Read/Write Control"("FPGA VI Reference In"=w3439, "error in"=w3438, "FPGA Trap Trig"=w3437) -> ("FPGA VI Reference Out"=w3436:T20, "error out"=w3435:errorcluster)
        n2691 = xnode "Read/Write Control"("FPGA VI Reference In"=w3436, "error in"=w3435, "TTrig?"=w3437) -> ()  [unwired: 2 out]
        n2692 = local write "Initializing"(FALSE ("Initializing")) -> ()
        n2693 = local write "Triggered"(FALSE ("Triggered")) -> ()
        n2694 = local write "Waiting"(FALSE ("Waiting")) -> ()
      }
    }
    n2695 = Not(x=w3109) -> (.not. x?=w3122:bool)
    n2696 = And(x="Trap Trig. Fl.", y=w3122) -> (x .and. y?=w3119:bool)
    n2697 = local read "Tether"() -> (w3247:bool)
    n2698 = Or(x=w3119, y="Reinitialize") -> (x .or. y?=w3105:bool)
    n2699 = feedback #23(w3115) -> (w3120:string)
    n2700 = Select(t=w3115, s=w3119, f=w3120) -> (s? t:f=w3114:string)
    n2701 = Select(t=w3115, s="Reinitialize", f=w3114) -> (s? t:f=w3113:string)
    n2702 = feedback #24(0) -> (w3117:i32)
    n2703 = feedback #25(w3240) -> (w3239:dbl[])
    n2704 = Build Array (concatenate)(w3240, w3239) -> (w3073:dbl[])
    n2705 = case "For determining if there is a tether still" shown="True" w3247 {
      tunnel: w3246 -> [_ w3563]
      frame False {
      }
      frame True {
        n2706 = Greater?(x="Lost Tether Alarm Threshold (pN)", y=w3563) -> (0:w3561:bool)
        n2707 = case shown="True" w3561 {
          frame False {
          }
          frame True {
            w3564 = FALSE ("Value (Signaling)")
            n2708 = flat-sequence {
              frame #0 {
                # "stop only if saving"
                n2709 = local read "Saving..."() -> (w3576:bool)
                n2710 = And(x=w3576, y="TA Cancel Save?") -> (x .and. y?=w3575:bool)
                n2711 = local write "Stop Saving"(w3575) -> ()
              }
              frame #1 {
                n2712 = case shown="True" "TA Green Off?" {
                  frame False {
                  }
                  frame True {
                    w3579 = FALSE ("Fl. Triggered...")
                    n2713 = local write "Fl. Triggered..."(w3579) -> ()
                    n2714 = property on="Green Laser ON" class="Bool (strict)"("Val(Sgnl)"=w3579) -> ()  [unwired: 2 in, 2 out]
                  }
                }
              }
            }
            n2715 = local read "Time tether formed"() -> (w3570:timestamp)
            n2716 = Get Date/Time In Seconds() -> (seconds since 1Jan1904=w3571:timestamp)
            n2717 = Subtract(x=w3571, y=w3570) -> (x-y=w3569:dbl)
            n2718 = Number To Decimal String(number=w3569) -> (decimal integer string=w3566:string)  [unwired: 1 out]
            n2719 = local read "Messages"() -> (w3573:string)
            n2720 = call <vilib>:"Beep.vi"() -> ()  [unwired: 3 in, 9 out]
            n2721 = Concatenate Strings("Lost tether (" ("Message to add"), w3566, " s)." ("string")) -> (w3568:string)
            n2722 = local write "Tether"(FALSE ("Tether")) -> ()
            n2723 = call "Update messages.vi"("Message to add"=w3568, "Old message string"=w3573) -> ("New message string"=w3572:string)
            n2724 = local write "Messages"(w3572) -> ()
            n2725 = property on="Fl. Triggered..." class="Bool (strict)"("Val(Sgnl)"=w3564) -> ()  [unwired: 2 in, 2 out]
            n2726 = local write "Dip for Protein"(w3564) -> ()
            n2727 = property on="Trap Pos. FB ON" class="Bool (strict)"("Val(Sgnl)"=w3564) -> ()  [unwired: 2 in, 2 out]
            n2728 = property on="Trap Trig. Fl." class="Bool (strict)"("Val(Sgnl)"=w3564) -> ()  [unwired: 2 in, 2 out]
          }
        }
      }
    }
    n2729 = case "For triggering actions based on the trap position (e.g., turning the excitation laser on if trap under feedback moves so far)" shown="True" "Trap Trig. Fl." {
      tunnel: w3100 -> [_ w3452]
      tunnel: w3113 -> [_ w3451]
      tunnel: ["" ("t") w3450] -> w3121
      tunnel: w3105 -> [_ w3449]
      tunnel: [0 ("t") w3448] -> w3118
      tunnel: w3117 -> [_ w3447]
      tunnel: w3092 -> [_ w3446]
      tunnel: w3091 -> [_ w3445]
      frame False {
      }
      frame True {
        n2730 = case shown="\"Wait for trigger\"" w3451 {
          tunnel: w3452 -> [w3469 _ _ w3517]
          tunnel: [w3466 w3498 "" ("t") w3520] -> w3450
          tunnel: w3449 -> [_ _ _ w3508]
          tunnel: [w3465 w3495 0 ("t") w3509] -> w3448
          tunnel: w3447 -> [_ w3497 _ w3515]
          tunnel: w3446 -> [w3454 w3492 _ w3511]
          tunnel: w3445 -> [w3453 w3491 _ w3510]
          frame "Wait for trigger" {
            n2731 = local read "Trap Trig. (FPGA)"() -> (w3457:bool)
            n2732 = Subtract(x=w3469, y="Mean T1 Position\nto compare (nm)") -> (x-y=w3462:dbl[])
            n2733 = call <vilib>:"Std Deviation and Variance.vi"("X"=w3462) -> ("mean"=→"mean":dbl, "standard deviation"=→"standard\ndeviation":dbl)  [unwired: 1 in, 1 out]
            n2734 = Array Max & Min(array=w3462) -> (max value=→"max value":dbl, min value=→"min value":dbl)  [unwired: 2 out]
            n2735 = Greater?(x=w3462, y="Threshold (nm)") -> (0:w3472:bool[])
            n2736 = case shown="True" w3457 {
              tunnel: w3454 -> [_ w3478]
              tunnel: w3453 -> [_ w3477]
              tunnel: [FALSE ("TTrig?") w3476] -> w3460
              frame False {
              }
              frame True {
                n2737 = xnode "Read/Write Control"("FPGA VI Reference In"=w3478, "error in"=w3477) -> ("TTrig?"=w3476:bool)  [unwired: 2 out]
              }
            }
            n2738 = Or Array Elements(Boolean array=w3472) -> (logical OR=w3459:bool)
            n2739 = Select(t=w3460, s=w3457, f=w3459) -> (s? t:f=w3458:bool)
            n2740 = Not(x=w3457) -> (.not. x?=w3456:bool)
            n2741 = And(x=w3458, y=w3456) -> (x .and. y?=w3455:bool)
            n2742 = Select(t="Triggered", s=w3458, f="Wait for trigger") -> (s? t:f=w3466:string)
            n2743 = case shown="True" w3458 {
              tunnel: [0 0] -> w3465
              tunnel: w3454 -> [_ w3483]
              tunnel: w3453 -> [_ w3482]
              frame False {
                "Waiting" <- TRUE ("Waiting")
              }
              frame True {
                n2744 = xnode "Read/Write Control"("FPGA VI Reference In"=w3483, "error in"=w3482, "TTrig?"=FALSE) -> ()  [unwired: 2 out]
                n2745 = local read "Messages"() -> (w3486:string)
                n2746 = call <vilib>:"Beep.vi"() -> ()  [unwired: 12 in]
                n2747 = call "Update messages.vi"("Message to add"="Unwinding trigger.", "Old message string"=w3486) -> ("New message string"=w3487:string)
                n2748 = local write "Messages"(w3487) -> ()
                n2749 = local write "Waiting"(FALSE ("Waiting")) -> ()
                "Triggered" <- TRUE ("Triggered")
              }
            }
            n2750 = case "Only need to turn on laser if host triggered" shown="True" w3455 {
              frame False {
              }
              frame True {
                n2751 = property on="Green Laser ON" class="Bool (strict)"("Val(Sgnl)"=TRUE ("Value (Signaling)")) -> ()  [unwired: 2 in, 2 out]
              }
            }
          }
          frame "Triggered" {
            n2752 = local read "Trap Trig. (FPGA)"() -> (w3494:bool)
            n2753 = Increment(x=w3497) -> (x+1=w3495:i32)
            n2754 = Greater Or Equal?(x=w3495, y="Fl. ON time (n)") -> (x >= y?=w3493:bool)
            n2755 = Select(t="Wait for trigger", s=w3493, f="Triggered" ("t")) -> (s? t:f=w3498:string)
            n2756 = And(x=w3493, y=w3494) -> (x .and. y?=w3490:bool)
            n2757 = case shown="True" w3490 {
              tunnel: w3492 -> [_ w3502]
              tunnel: w3491 -> [_ w3501]
              frame False {
              }
              frame True {
                n2758 = xnode "Read/Write Control"("FPGA VI Reference In"=w3502, "error in"=w3501, "FPGA Trap Trig"=TRUE) -> ()  [unwired: 2 out]
              }
            }
            n2759 = case shown="True" w3493 {
              frame False {
              }
              frame True {
                w3504 = FALSE ("Value (Signaling)")
                n2760 = local write "Triggered"(w3504) -> ()
                n2761 = local write "Waiting"(TRUE ("Waiting")) -> ()
                n2762 = property on="Green Laser ON" class="Bool (strict)"("Val(Sgnl)"=w3504) -> ()  [unwired: 2 in, 2 out]
              }
            }
          }
          frame "Do nothing" {
          }
          frame "Initialize", Default {
            n2763 = Increment(x=w3515) -> (x+1=w3519:i32)
            n2764 = Select(t=1, s=w3508, f=w3519) -> (s? t:f=w3509:i32)
            n2765 = feedback #26(w3517) -> (w3523:dbl[])
            n2766 = Build Array (concatenate)(w3517, w3523) -> (w3516:dbl[])
            n2767 = Greater Or Equal?(x=w3509, y="Wait to get offset (n)") -> (x >= y?=w3512:bool)
            n2768 = Select(t=w3517, s=w3508, f=w3516) -> (s? t:f=w3518:dbl[])
            n2769 = feedback-in #26(w3518) -> ()
            n2770 = call-poly <vilib>:"Mean.vi"("X"=w3518) -> ("mean"=w3513:dbl)  [unwired: 1 out]
            n2771 = local write "Mean T1 Position\nto compare (nm)"(w3513) -> ()
            n2772 = case shown="True" w3508 {
              tunnel: w3511 -> [_ w3529]
              tunnel: w3510 -> [_ w3528]
              frame False {
              }
              frame True {
                w3525 = FALSE ("FPGA Trap Trig")
                n2773 = xnode "Read/Write Control"("FPGA VI Reference In"=w3529, "error in"=w3528, "FPGA Trap Trig"=w3525) -> ("FPGA VI Reference Out"=w3527:T20, "error out"=w3526:errorcluster)
                n2774 = xnode "Read/Write Control"("FPGA VI Reference In"=w3527, "error in"=w3526, "TTrig?"=w3525) -> ()  [unwired: 2 out]
              }
            }
            n2775 = Select(t="Wait for trigger", s=w3512, f="Initialize") -> (s? t:f=w3520:string)
            n2776 = case shown="True" w3512 {
              tunnel: w3513 -> [_ w3532]
              tunnel: w3511 -> [_ w3541]
              tunnel: w3510 -> [_ w3540]
              frame False {
                n2777 = local write "Waiting"(FALSE ("Waiting")) -> ()
                "Initializing" <- TRUE ("Initializing")
              }
              frame True {
                n2778 = local read "Threshold (nm)"() -> (w3544:dbl)
                n2779 = local read "AOM X Cal (nm/MHz)"() -> (w3543:dbl)
                n2780 = Add(x=w3532, y=w3544) -> (x+y=w3545:dbl)
                n2781 = Divide(x=w3545, y=w3543) -> (x/y=w3542:dbl)
                n2782 = call "IR AOM freq to word.vi"("Frequency In (MHz)"=w3542) -> ("Frequency Word Out (double)"=w3539:dbl)
                n2783 = local write "Initializing"(FALSE ("Initializing")) -> ()
                n2784 = local write "Waiting"(TRUE ("Waiting")) -> ()
                n2785 = To Quad Integer(1:w3539) -> (0:w3538:i64)
                n2786 = xnode "Read/Write Control"("FPGA VI Reference In"=w3541, "error in"=w3540, "FPGA TTrig Thresh"=w3538) -> ("FPGA VI Reference Out"=w3535:T20, "error out"=w3534:errorcluster)
                n2787 = xnode "Read/Write Control"("FPGA VI Reference In"=w3535, "error in"=w3534, "FPGA Trap Trig"=TRUE) -> ()  [unwired: 2 out]
              }
            }
          }
        }
      }
    }
    n2788 = feedback-in #23(w3121) -> ()
    n2789 = feedback-in #24(w3118) -> ()
    n2790 = Split 1D Array(array=w3073, index=w3135) -> (first subarray=w3236:dbl[])  [unwired: 1 out]
    n2791 = feedback-in #25(w3236) -> ()
    n2792 = call-poly <vilib>:"Mean.vi"("X"=w3236) -> ("mean"=w3235:dbl)  [unwired: 1 out]
    "Bead Mean (nm)" <- w3235
    n2793 = Subtract(x=w3236, y=w3235) -> (x-y=w3234:dbl[])
    n2794 = Square(x=w3234) -> (x^2=w3233:dbl[])
    n2795 = call-poly <vilib>:"Mean.vi"("X"=w3233) -> ("mean"=w3232:dbl)  [unwired: 1 out]
    n2796 = Square Root(x=w3232) -> (sqrt(x)=w3231:dbl)
    n2797 = Multiply(x=10.0, y=w3231) -> (x*y=→"RMS (Ang)":dbl)
